vi "ReadAndWriteFile.vi"   [LabVIEW 2014]
types:
  T1 = enum16{"open", "replace", "create", "open or create", "replace or create", "replace or create with confirmation"}
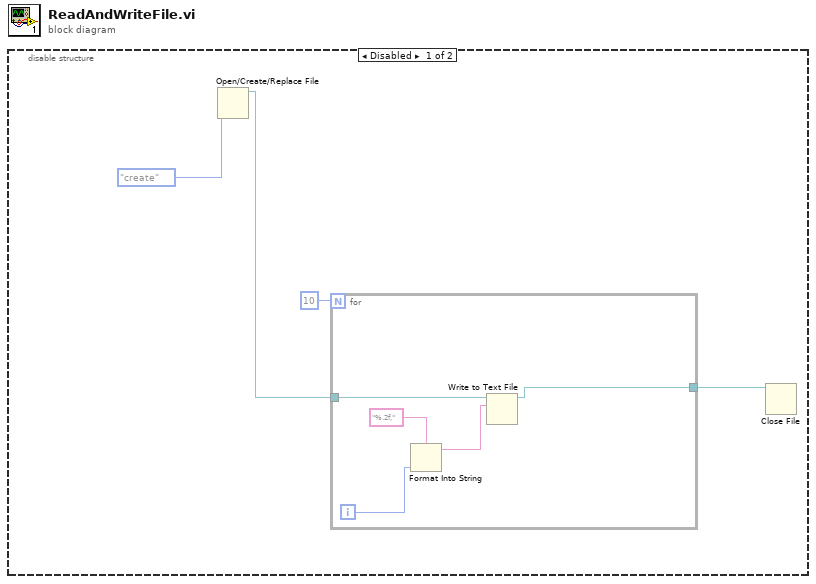
[diagram p0: block diagram]
diagram:
  n1 = disable-structure shown="Disabled" {
    frame Disabled {
      n2 = Open/Create/Replace File(operation (0:open)=T1."create") -> (refnum out=w2:refnum<file>)  [unwired: 5 in, 2 out]
      n3 = for {
        N: 10 -> [_]
        tunnel: w2 -> [w9]
        tunnel: [w6] -> w1
        i -> [w8]
        n4 = Format Into String(format string="%.2f,", w8) -> (resulting string=w7:string)  [unwired: 2 in, 1 out]
        n5 = Write to Text File(file (use dialog)=w9, text=w7) -> (refnum out=w6:refnum<file>)  [unwired: 2 in, 2 out]
      }
      n6 = Close File(refnum=w1) -> ()  [unwired: 1 in, 2 out]
    }
    frame Enabled {
    }
  }
